vi "Translate Menu Strings.vi"(8 "error in (no error)":errorcluster, 9 "Language Index (0)":i32, 10 "Preview?":bool, 11 "Menu Data in":refnum<class "Menu Data.lvclass">) -> (0 "error out":errorcluster, 2 "Preview Path out":path, 3 "Menu Data out":refnum<class "Menu Data.lvclass">)   [LabVIEW 2013, in "SET Project Data.lvlib" / "Menu Data.lvclass"]
uses:
  Menu Data.lvclass
  Menu Data.lvclass/Menu Data.ctl
  Resource Data Class/Resource Data.lvclass
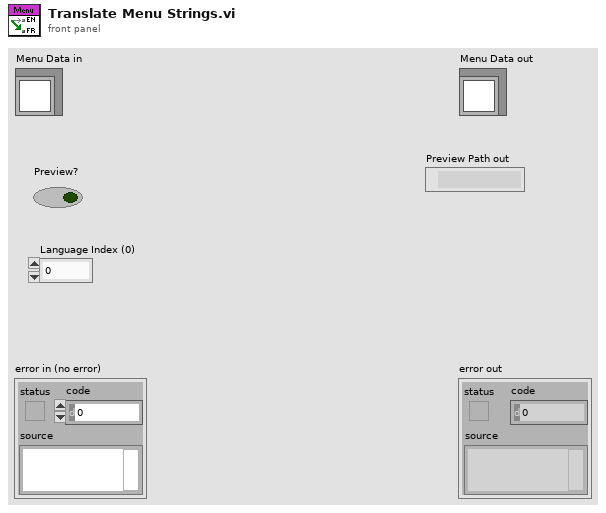
[diagram p1: front panel]
types:
  T1 = enum32{"Invalid", "Standard", "Closed", "Hidden", "Minimized", "Maximized"}
  T2 = typedef "LVMenuShortCut.ctl" = cluster{"include Shift key?":bool, "include Ctrl key?":bool, "shortcut key":string}
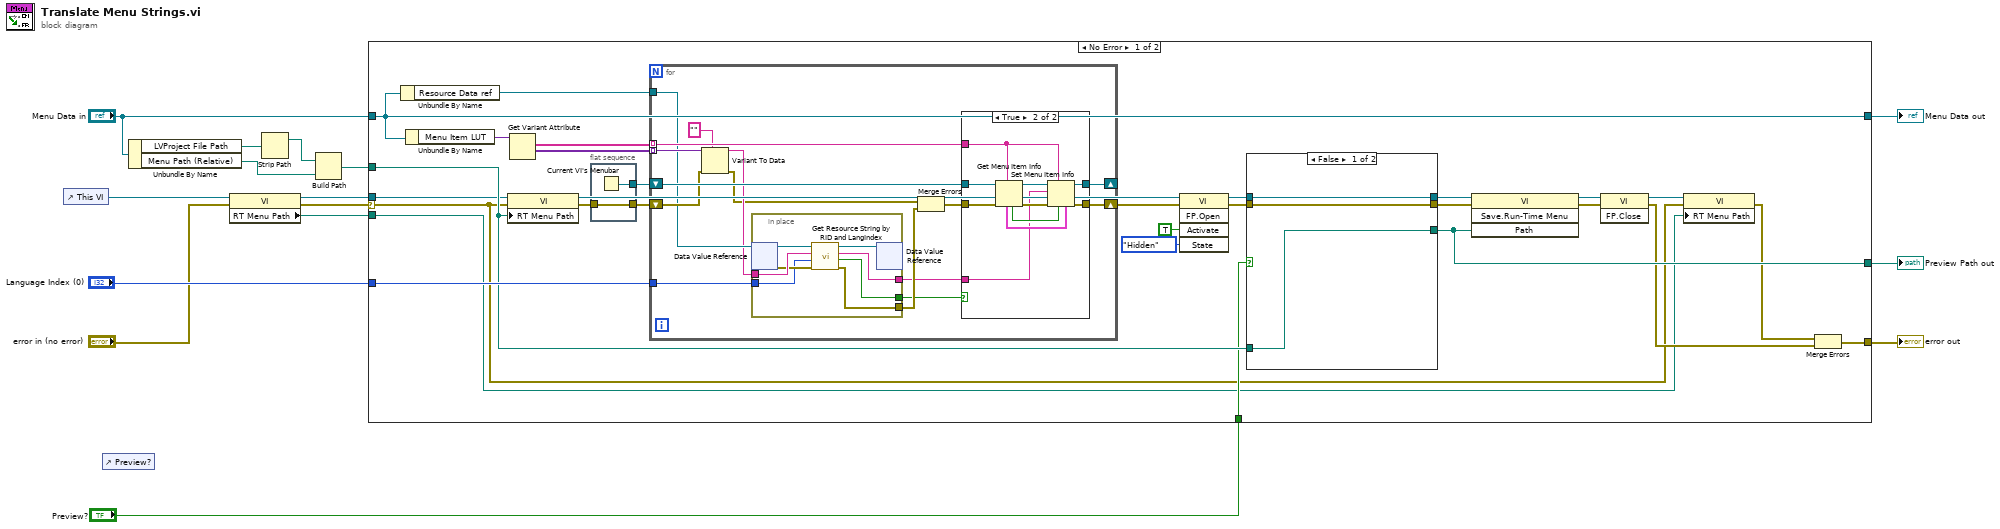
[diagram p0: block diagram]
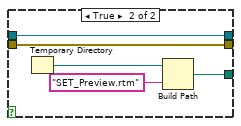
[diagram p2: hidden frame]
diagram:
  n1 = control-ref of="This VI"() -> (w5:refnum<vi>)
  n2 = control-ref of="Preview?"() -> ()  [unwired: 1 out]
  n3 = Unbundle By Name("Menu Data in") -> ("LVProject File Path"=w11:path, "Menu Path (Relative)"=w13:path)
  n4 = property class="VI"(reference=w5, error in="error in (no error)") -> (reference out=w4:refnum<vi>, error out=w2:errorcluster, "RT Menu Path"=w1:path)
  n5 = Strip Path(path=w11) -> (stripped path=w12:path)  [unwired: 1 out]
  n6 = Build Path(base path=w12, name or relative path=w13) -> (appended path=w9:path)
  n7 = case shown="No Error" w2 {
    selector: w2 -> [w17 w92]
    tunnel: [w19 w92] -> w15
    tunnel: [w37 w91] -> w14
    tunnel: "Menu Data in" -> [w37 w91]
    tunnel: w9 -> [w35 _]
    tunnel: "Language Index (0)" -> [w38 _]
    tunnel: "Preview?" -> [w34 _]
    tunnel: [w24 _] -> w6
    tunnel: w4 -> [w18 _]
    tunnel: w1 -> [w16 _]
    frame No Error {
      n8 = Unbundle By Name(w37) -> ("Resource Data ref"=w36:refnum<data-value>)
      n9 = Unbundle By Name(w37) -> ("Menu Item LUT"=w41:variant)
      n10 = property class="VI"(reference=w18, error in=w17, "RT Menu Path"=w35) -> (reference out=w31:refnum<vi>, error out=w44:errorcluster)
      n11 = Get Variant Attribute(Variant=w41) -> (names=w40:string[], values=w39:variant[])  [unwired: 3 in, 2 out]
      n12 = flat-sequence {
        tunnel: [w90] -> w43
        tunnel: w44 -> [w89]
        tunnel: [w89] -> w42
        frame #0 {
          n13 = Current VI's Menubar() -> (w90:refnum<k9>)
        }
      }
      n14 = for {
        tunnel: w40 -> [w65] mode=indexing
        shift-right: [w66] -> w29
        shift-left: w42 -> [w62]
        tunnel: w39 -> [w64] mode=indexing
        tunnel: w38 -> [w60]
        tunnel: w36 -> [w61]
        shift-right: [w53] -> _
        shift-left: w43 -> [w67]
        n15 = Variant To Data(error in=w62, type="", Variant=w64) -> (data=w59:string, error out=w58:errorcluster)
        n16 = in-place {
          in-place-border: w59 -> [w86]
          in-place-border: [w84] -> w54
          in-place-border: [w83] -> w57
          in-place-border: w60 -> [w82]
          in-place-border: [w81] -> w55
          n17 = in-place-dvr #1(w61) -> (w88:refnum<class "Resource Data.lvclass">, w85:errorcluster)
          n18 = call "Get Resource String by RID and LangIndex.vi"("error in (no error)"=w85, "LangIndex (0)"=w82, "RID"=w86, "LangFile in"=w88) -> ("error out"=w83:errorcluster, "Found?"=w84:bool, "Translated Text (ASCII)"=w81:string, "LangFile out"=w87:refnum<class "Resource Data.lvclass">)  [unwired: 4 in]
          n19 = in-place-dvr #1(w87) -> ()  [unwired: 2 out]
        }
        n20 = Merge Errors(w58, w57) -> (w56:errorcluster)
        n21 = case shown="True" w54 {
          tunnel: w67 -> [w68 w80]
          tunnel: [w69 w75] -> w66
          tunnel: w65 -> [_ w74]
          tunnel: w56 -> [w69 w72]
          tunnel: w55 -> [_ w71]
          tunnel: [w68 w70] -> w53
          frame False {
          }
          frame True {
            n22 = Get Menu Item Info(7:w74, 8:w72, 11:w80) -> (0:w78:errorcluster, 1:w73:bool, 3:w79:refnum<k9>, 4:w76:bool, 6:w77:T2)  [unwired: 2 out]
            n23 = Set Menu Item Info(4:w77, 6:w76, 7:w74, 8:w78, 9:w73, 10:w71, 11:w79) -> (0:w75:errorcluster, 3:w70:refnum<k9>)
          }
        }
      }
      n24 = invoke class="VI" method="FP.Open"(reference=w31, error in=w29, "Activate"=TRUE ("Activate?"), "State"=T1."Hidden") -> (reference out=w30:refnum<vi>, error out=w28:errorcluster)  [unwired: 1 in, 3 out]
      n25 = case shown="False" w34 {
        tunnel: w28 -> [w45 w52]
        tunnel: w30 -> [w46 w50]
        tunnel: [w45 w52] -> w23
        tunnel: w35 -> [w47 _]
        tunnel: [w47 w51] -> w24
        tunnel: [w46 w50] -> w26
        frame False {
        }
        frame True {
          n26 = Temporary Directory() -> (w49:path)
          n27 = Build Path(base path=w49, name or relative path="SET_Preview.rtm") -> (appended path=w51:path)
        }
      }
      n28 = invoke class="VI" method="Save.Run-Time Menu"(reference=w26, error in=w23, "Path"=w24) -> (reference out=w25:refnum<vi>, error out=w22:errorcluster)  [unwired: 1 in, 2 out]
      n29 = invoke class="VI" method="FP.Close"(reference=w25, error in=w22) -> (reference out=w27:refnum<vi>, error out=w20:errorcluster)  [unwired: 1 in, 1 out]
      n30 = property class="VI"(reference=w27, error in=w17, "RT Menu Path"=w16) -> (error out=w21:errorcluster)  [unwired: 1 out]
      n31 = Merge Errors(w21, w20) -> (w19:errorcluster)
    }
    frame Error {
    }
  }
  "error out" <- w15
  "Menu Data out" <- w14
  "Preview Path out" <- w6
